vi "PQescapeBytea.vi"(8 "error in (no error)":errorcluster, 9 "to_length":u64, 10 "from_length":u64, 11 "from":string) -> (0 "error out":errorcluster, 2 "PQescapeBytea":string, 3 "to_length out":u64)   [LabVIEW 2019, in "libpqlv64.lvlib"]
uses:
  libpqlv64.lvlib
  libpq.dll
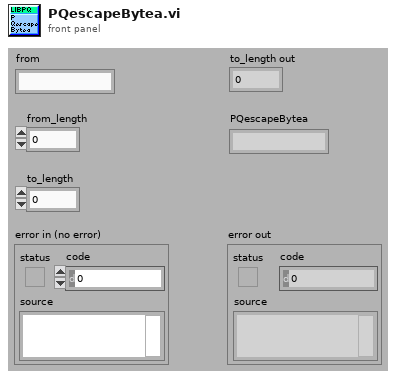
[diagram p1: front panel]
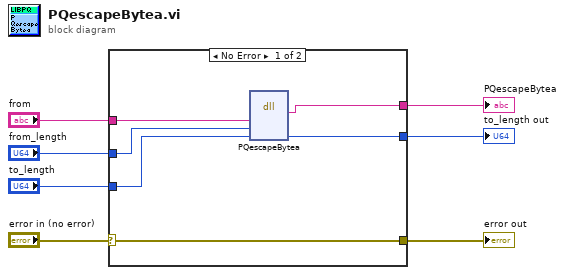
[diagram p0: block diagram]
diagram:
  n1 = case shown="No Error" "error in (no error)" {
    selector: "error in (no error)" -> [w13 w15]
    tunnel: [w13 w15] -> w6
    tunnel: [w12 _] -> w5
    tunnel: "from" -> [w11 _]
    tunnel: "from_length" -> [w10 _]
    tunnel: "to_length" -> [w9 w14]
    tunnel: [w8 w14] -> w1
    frame No Error {
      n2 = dll-call lib="libpq.*" fn="PQescapeBytea"("from"=w11, "from_length"=w10, "to_length"=w9) -> ("return type"=w12:string, "to_length"=w8:u64)  [unwired: 5 in, 2 out]
    }
    frame Error {
    }
  }
  "PQescapeBytea" <- w5
  "to_length out" <- w1
  "error out" <- w6
